vi "sub1.vi"(10 "regular expression":string, 11 "Array":T1(array[cluster])) -> (3 "Tunnel out":refnum<vi>)   [LabVIEW 2020, in "CSM-Helper.lvclass"]
uses:
  CSM-Helper.lvclass
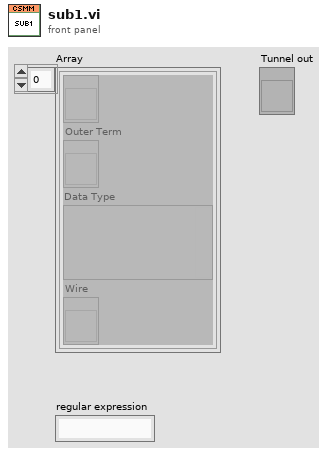
[diagram p1: front panel]
types:
  T1 = cluster{refnum<vi>, "Outer Term":refnum<vi>, "Data Type":variant, "Wire":refnum<vi>}[]
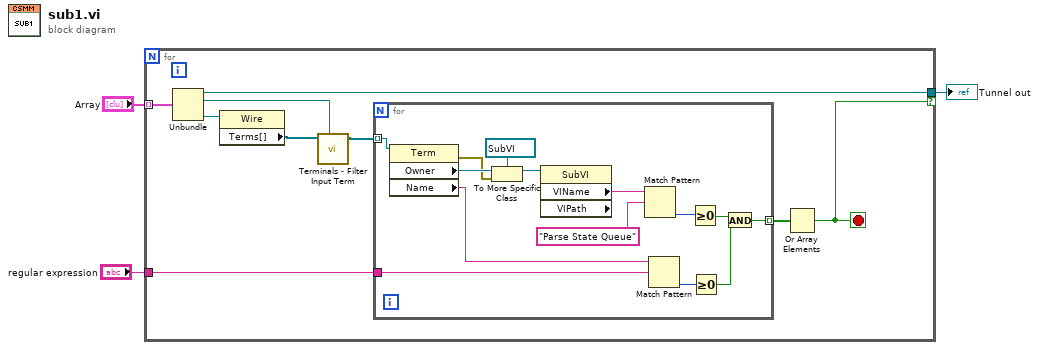
[diagram p0: block diagram]
diagram:
  n1 = for {
    tunnel: "Array" -> [w12] mode=indexing
    tunnel: [w10] -> w2 if=w7
    tunnel: "regular expression" -> [w8]
    stop <- w7 stop-if-true
    n2 = Unbundle(w12) -> (w10:refnum<vi>, "Outer Term"=w4:refnum<vi>, "Wire"=w11:refnum<vi>)  [unwired: 1 out]
    n3 = property class="Wire"(reference=w11) -> ("Terms[]"=w6:refnum<vi>[])  [unwired: 1 in, 2 out]
    n4 = call "Terminals - Filter Input Term.vi"("InnerTerminal in"=w4, "Wire.Terms[] in"=w6) -> ("Wire.Terms[] out"=w5:refnum<vi>[])  [unwired: 9 in]
    n5 = for {
      tunnel: [w15] -> w9 mode=indexing
      tunnel: w8 -> [w14]
      tunnel: w5 -> [w13] mode=indexing
      n6 = property class="Term"(reference=w13) -> (error out=w24:errorcluster, "Owner"=w26:refnum<vi>, "Name"=w20:string)  [unwired: 1 in, 1 out]
      n7 = To More Specific Class(target class=refnum<vi> refnum ("Parse State Queue"), reference=w26, error in=w24) -> (specific class reference=w23:refnum<vi>)  [unwired: 1 out]
      n8 = property class="SubVI" props=["VIName", "VIPath"](reference=w23) -> ("VIName"=w22:string)  [unwired: 1 in, 3 out]
      n9 = Match Pattern(string=w22, regular expression="Parse State Queue") -> (offset past match=w19:i32)  [unwired: 1 in, 3 out]
      n10 = Match Pattern(string=w20, regular expression=w14) -> (offset past match=w18:i32)  [unwired: 1 in, 3 out]
      n11 = Greater Or Equal To 0?(x=w19) -> (x >= 0?=w17:bool)
      n12 = Greater Or Equal To 0?(x=w18) -> (x >= 0?=w16:bool)
      n13 = And(x=w17, y=w16) -> (x .and. y?=w15:bool)
    }
    n14 = Or Array Elements(Boolean array=w9) -> (logical OR=w7:bool)
  }
  "Tunnel out" <- w2
